vi "Get ao_parameter.vi"(11 "MulticolumnListbox in":refnum<vi>) -> (2 "Output_Value":dbl[](array[numeric]), 3 "Channel name":string[](array[string]))   [LabVIEW 2017]
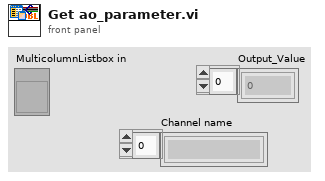
[diagram p1: front panel]
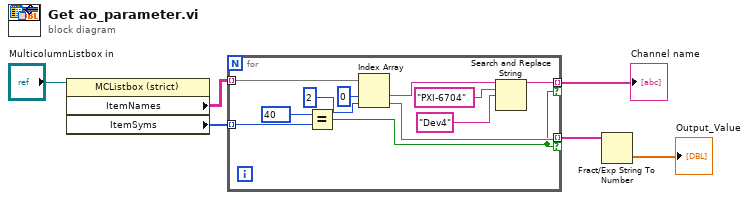
[diagram p0: block diagram]
diagram:
  n1 = property on="Property Node" class="MCListbox (strict)"(reference="MulticolumnListbox in") -> ("ItemNames"=w6:string[][], "ItemSyms"=w5:i32[])  [unwired: 1 in, 2 out]
  n2 = for {
    tunnel: w5 -> [w16] mode=indexing
    tunnel: w6 -> [w15] mode=indexing
    tunnel: [w9] -> w1 mode=indexing if=w7
    tunnel: [w8] -> w3 mode=indexing if=w7
    n3 = Equal?(x=40, y=w16) -> (x = y?=w7:bool)
    n4 = Index Array(array=w15, index #1=0, index #2=2) -> (element #1=w12:string, element #2=w8:string)
    n5 = Search and Replace String(input string=w12, search string="PXI-6704", replace string="Dev4") -> (result string=w9:string)  [unwired: 5 in, 3 out]
  }
  "Channel name" <- w1
  n6 = Fract/Exp String To Number(string=w3) -> (number=→"Output_Value":dbl[])  [unwired: 3 in, 1 out]
